vi "Utility Create Batch Launcher for Exe.vi"(6 "Enable (T)":bool=TRUE, 8 "error in (no error)":errorcluster, 9 "Files Generated by Build":path[](array[path]), 10 "Build Specification Name":string, 11 "Extra Destination Copy":path) -> (0 "error out":errorcluster)   [LabVIEW 2015]
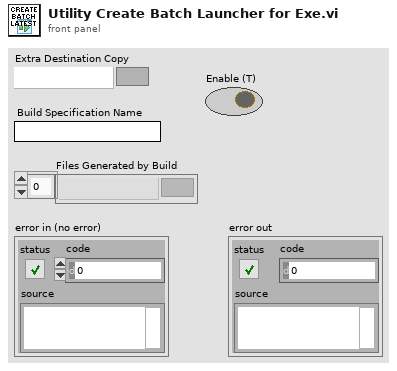
[diagram p1: front panel]
types:
  T1 = enum16{"open", "replace", "create", "open or create", "replace or create", "replace or create with confirmation"}
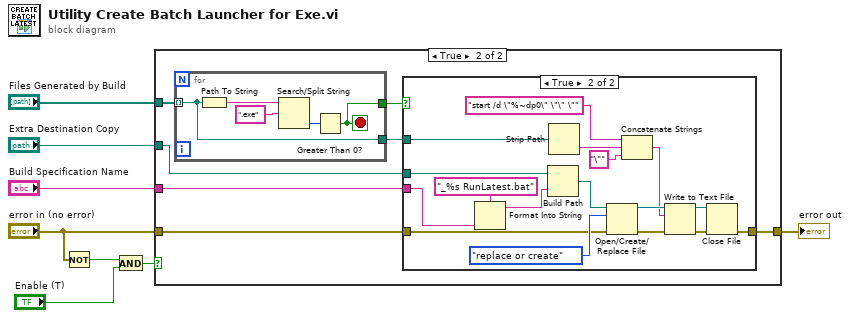
[diagram p0: block diagram]
diagram:
  n1 = Not(x="error in (no error)") -> (.not. x?=w2:bool)
  n2 = And(x=w2, y="Enable (T)") -> (x .and. y?=w4:bool)
  n3 = case shown="True" w4 {
    tunnel: [w9 w16] -> w8
    tunnel: "Build Specification Name" -> [_ w15]
    tunnel: "Extra Destination Copy" -> [_ w14]
    tunnel: "Files Generated by Build" -> [_ w11]
    tunnel: "error in (no error)" -> [w9 w10]
    frame False {
    }
    frame True {
      n4 = for {
        tunnel: w11 -> [w35] mode=indexing
        tunnel: [w36] -> w12
        tunnel: [w35] -> w13
        stop <- w36 stop-if-true
        n5 = Path To String(path=w35) -> (string=w39:string)
        n6 = Search/Split String(string=w39, search string/char (-)=".exe" ("regular expression")) -> (offset of match=w37:i32)  [unwired: 1 in, 2 out]
        n7 = Greater Than 0?(x=w37) -> (x > 0?=w36:bool)
      }
      n8 = case shown="True" w12 {
        tunnel: w13 -> [_ w34]
        tunnel: w14 -> [_ w32]
        tunnel: w15 -> [_ w19]
        tunnel: w10 -> [w17 w30]
        tunnel: [w17 w25] -> w16
        frame False {
        }
        frame True {
          n9 = Format Into String(format string="_%s RunLatest.bat" ("string"), w19) -> (resulting string=w18:string)  [unwired: 2 in, 1 out]
          n10 = Build Path(base path=w32, name or relative path=w18) -> (appended path=w31:path)
          n11 = Strip Path(path=w34) -> (name=w24:string)  [unwired: 1 out]
          n12 = Open/Create/Replace File(file path (use dialog)=w31, error in=w30, operation (0:open)=T1."replace or create") -> (refnum out=w28:refnum<file>, error out=w29:errorcluster)  [unwired: 3 in, 1 out]
          n13 = Concatenate Strings("start /d \"%~dp0\" \"\" \"" ("string"), w24, "\"" ("string")) -> (w21:string)
          n14 = Write to Text File(file (use dialog)=w28, text=w21, error in=w29) -> (refnum out=w26:refnum<file>, error out=w27:errorcluster)  [unwired: 1 in, 1 out]
          n15 = Close File(refnum=w26, error in=w27) -> (error out=w25:errorcluster)  [unwired: 1 out]
        }
      }
    }
  }
  "error out" <- w8
